vi "test harness_FXP_L_ye_Bend_u_singleAxis.vi"(8 "error in (no error)":errorcluster, 11 "TestCase in":refnum<class "FXP_observer_TestCase.lvclass">) -> (0 "error out":errorcluster, 3 "TestCase out":refnum<class "FXP_observer_TestCase.lvclass">)   [LabVIEW 2017, in "FXP_observer_TestCase.lvclass"]
uses:
  FXP_observer_TestCase.lvclass
  <vilib>/rvi/DesktopExecutionNode/Execution/niFpgaDEN_Execute.vi
  <vilib>/rvi/DesktopExecutionNode/DesktopExecutionNode.xnode
  <vilib>/addons/_JKI Toolkits/VI Tester/TestCase.llb/TestCase.lvclass
  C:/Program Files (x86)/National Instruments/LabVIEW 2017/vi.lib/addons/_JKI Toolkits/VI Tester/TestCase.llb/TestCase.lvclass
panel:
  out "x+y":fxp<+/-,51,11>[](array[numeric])
  out "xk_1_1":fxp<+/-,32,5>[](array[numeric])
  out "error (x_1_1)":errorcluster
  out "error (xu)":errorcluster
  out "error (yd)":errorcluster
  in  "x_u(k)":fxp<+/-,32,8>=13.600000023841858
  in  "Bz":fxp<+/-,32,5>[](array[numeric])=[1.0, 0.5, 0.20000000298023224, 0.20000000298023224, 0.29999999701976776, 2.0, 0.0, 0.0, 0.0, 0.0, 0.0, 0.0, 0.0, 0.0, 0.0, 0.0, 0.0, 0.0, 0.0, 0.0, 0.0, 0.0, 0.0, 0.0, 0.0, 0.0, 0.0, 0.0, 0.0, 0.0, 0.0, 0.0, 0.0, 0.0, 0.0, 0.0, 0.0, 0.0, 0.0, 0.0, 0.0, 0.0, 0.0, 0.0, 0.0, 0.0, 0.0, 0.0, 0.0, 0.0]
  in  "U(k): ux":fxp<+/-,18,5>=0.14501953125
  in  "y(k)":fxp<+/-,18,5>=0.123046875
  in  "NS":u8=5
  in  "Ldist":fxp<+/-,32,5>[](array[numeric])=[1.0, 0.5, 0.20000000298023224, 0.20000000298023224, 0.29999999701976776, 2.0, 0.0, 0.0, 0.0, 0.0, 0.0, 0.0, 0.0, 0.0, 0.0, 0.0, 0.0, 0.0, 0.0, 0.0, 0.0, 0.0, 0.0, 0.0, 0.0, 0.0, 0.0, 0.0, 0.0, 0.0, 0.0, 0.0, 0.0, 0.0, 0.0, 0.0, 0.0, 0.0, 0.0, 0.0, 0.0, 0.0, 0.0, 0.0, 0.0, 0.0, 0.0, 0.0, 0.0, 0.0]
  in  "x":fxp<+/-,32,5>[](array[numeric])=[1.0, 2.0, 3.0, 4.0, 5.0, 2.0, 0.0, 0.0, 0.0, 0.0, 0.0, 0.0, 0.0, 0.0, 0.0, 0.0, 0.0, 0.0, 0.0, 0.0, 0.0, 0.0, 0.0, 0.0, 0.0, 0.0, 0.0, 0.0, 0.0, 0.0, 0.0, 0.0, 0.0, 0.0, 0.0, 0.0, 0.0, 0.0, 0.0, 0.0, 0.0, 0.0, 0.0, 0.0, 0.0, 0.0, 0.0, 0.0, 0.0, 0.0]
  # "Remember that Ldist and Bz only have\ntwo integer bits!"
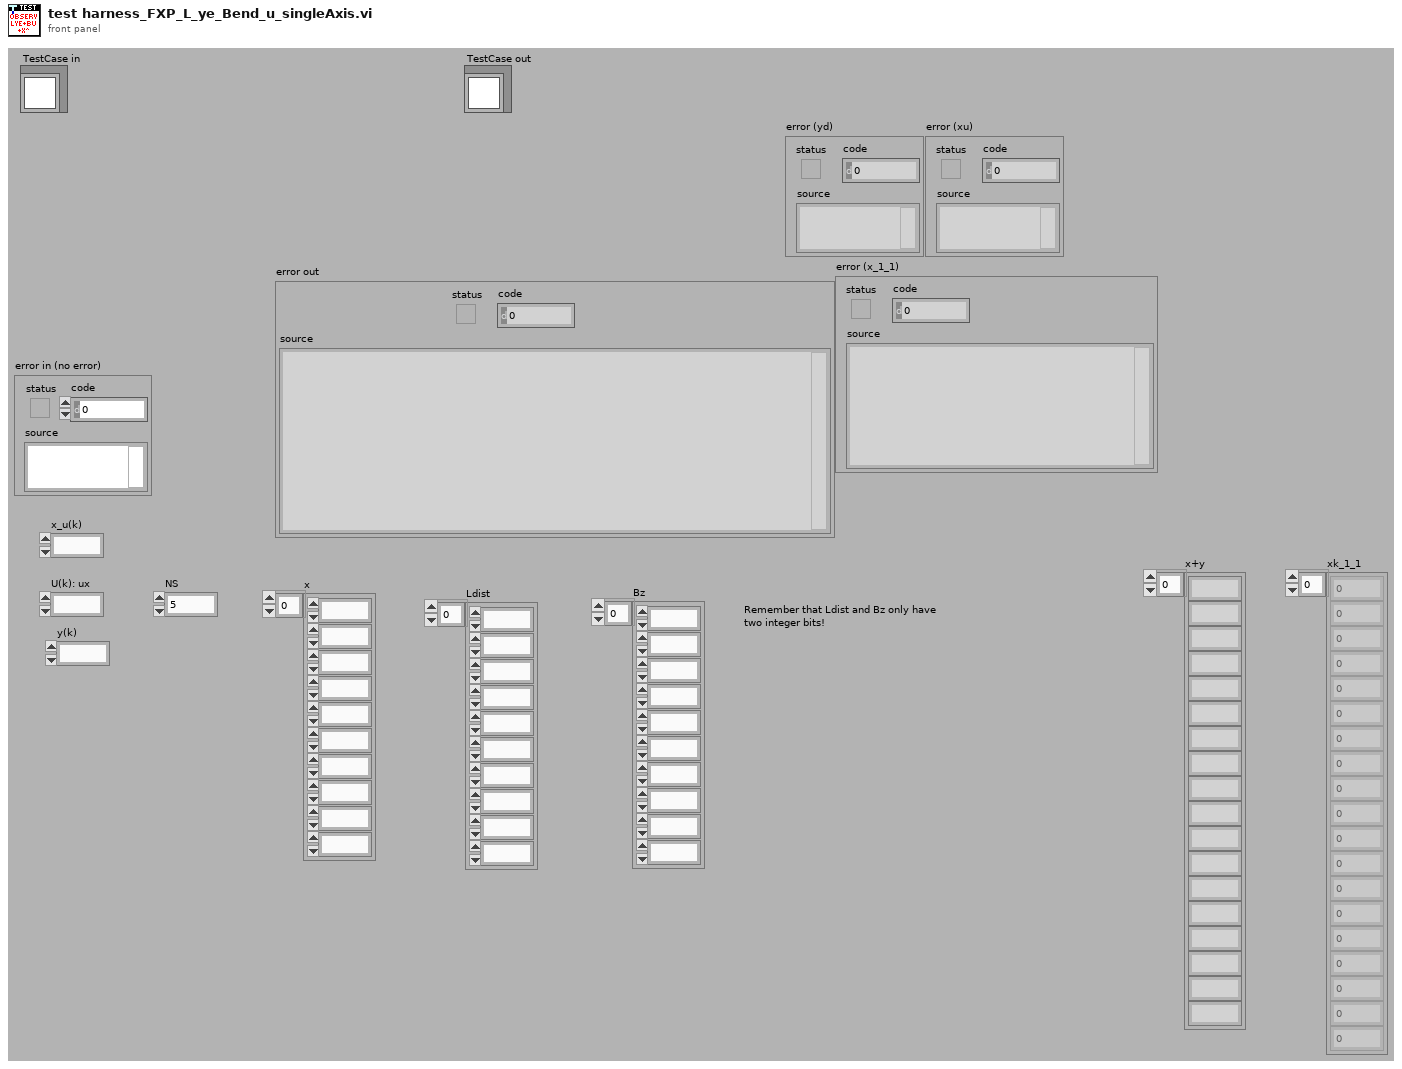
[diagram p1: front panel]
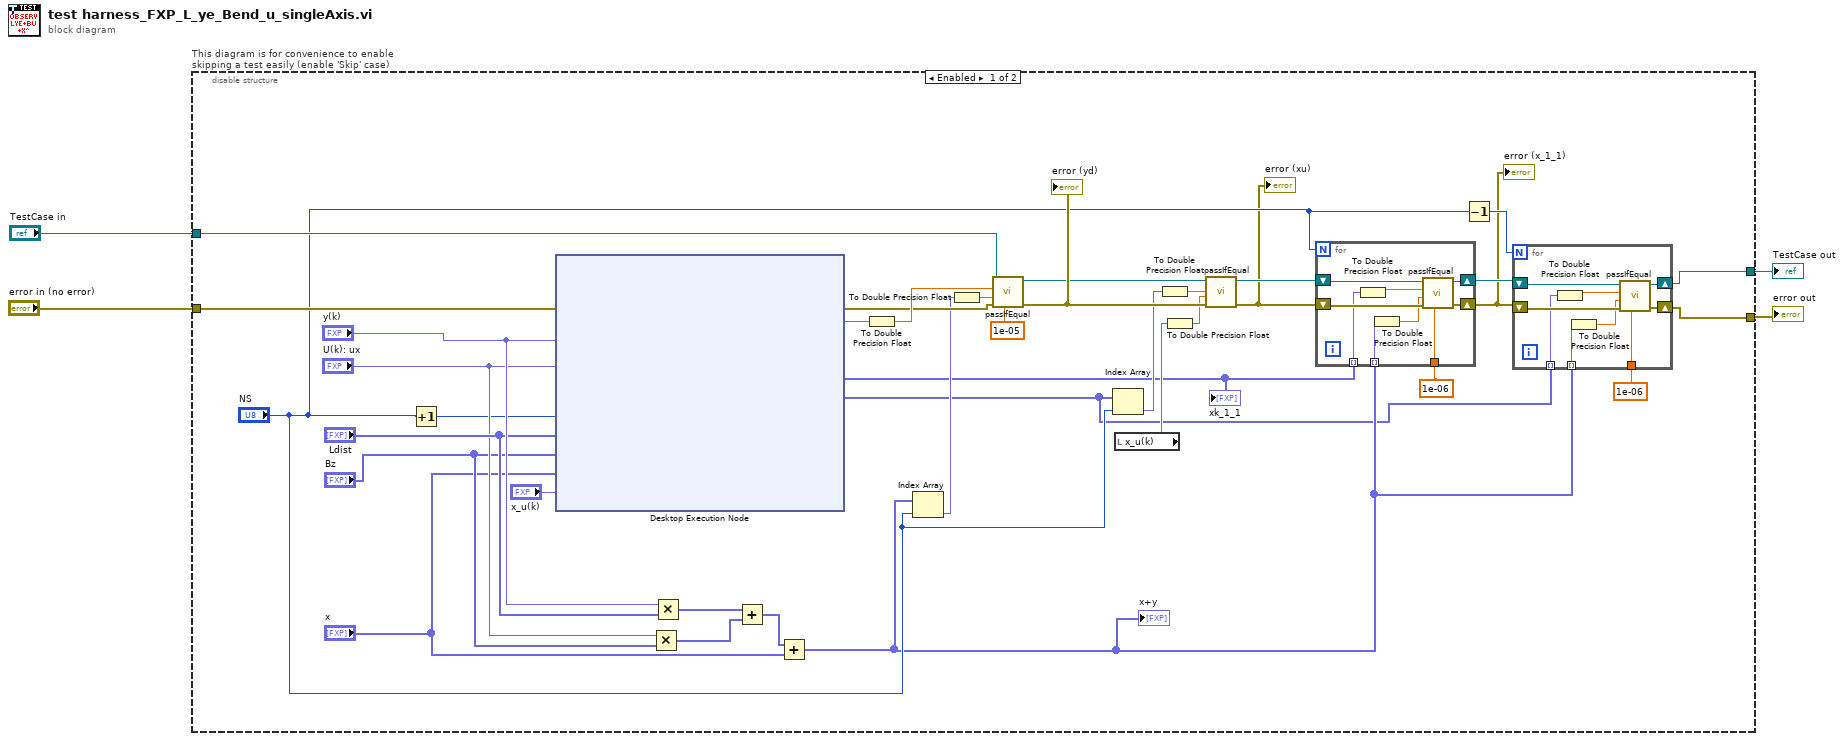
[diagram p0: block diagram]
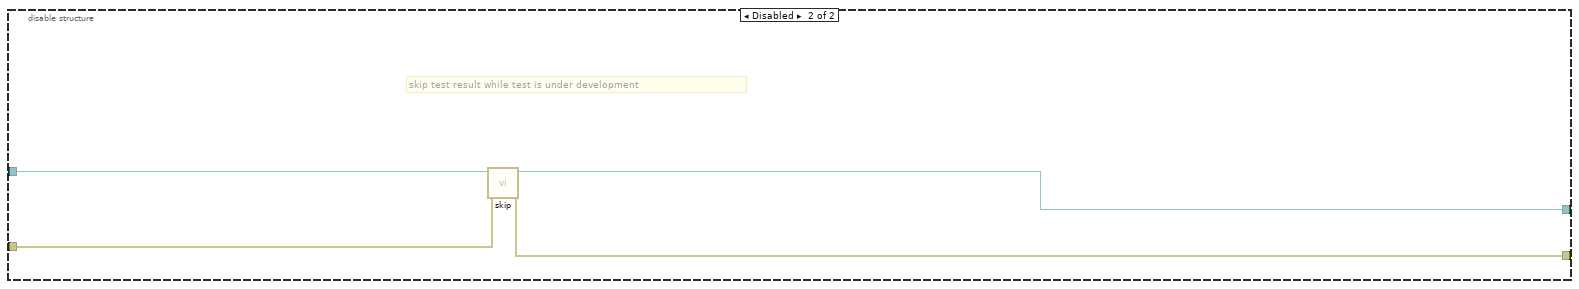
[diagram p2: hidden frame]
diagram:
  n1 = disable-structure "This diagram is for convenience to enable skipping a test easily (enable 'Skip' case)" shown="Enabled" {
    disable-tunnel: "TestCase in" -> [w41 w63]
    disable-tunnel: [w13 w61] -> w1
    disable-tunnel: [w12 w62] -> w3
    disable-tunnel: "error in (no error)" -> [w37 w60]
    frame Enabled {
      n2 = Increment(x="NS") -> (x+1=w25:u8)
      n3 = xnode "Desktop Execution Node"("Error In"=w37, "y(k)"="y(k)", "U(k): ux"="U(k): ux", "NS + 1"=w25, "Ldist"="Ldist", "Bz"="Bz", "x"="x", "x_u(k)"="x_u(k)") -> ("Error Out"=w38:errorcluster, "yd_est"=w28:fxp<+/-,32,5>, "xk_1_1"=w16:fxp<+/-,32,5>[], "xk_1_2"=w7:fxp<+/-,32,5>[])
      "xk_1_1" <- w16
      n4 = Multiply(x="U(k): ux", y="Bz") -> (x*y=w31:fxp<+/-,50,10>[])
      n5 = Multiply(x="y(k)", y="Ldist") -> (x*y=w32:fxp<+/-,50,10>[])
      n6 = Add(x=w32, y=w31) -> (x+y=w30:fxp<+/-,51,11>[])
      n7 = Add(x=w30, y="x") -> (x+y=w8:fxp<+/-,51,11>[])
      "x+y" <- w8
      n8 = To Double Precision Float(number=w28) -> (double precision float=w39:dbl)
      n9 = Index Array(array=w8, index="NS") -> (element=w26:fxp<+/-,51,11>)
      n10 = To Double Precision Float(number=w26) -> (double precision float=w27:dbl)
      n11 = call-dynamic "passIfEqual.vi"("delta (optional)"=1e-05 ("del u_x"), "error in (no error)"=w38, "y"=w27, "x"=w39, "TestCase in"=w41) -> ("error out"=w23:errorcluster, "TestCase out"=w22:refnum<class "FXP_observer_TestCase.lvclass">)  [unwired: 5 in]
      "error (yd)" <- w23
      n12 = Index Array(array=w7, index="NS") -> (element=w20:fxp<+/-,32,5>)
      n13 = local read "x_u(k)"() -> (w18:fxp<+/-,32,8>)
      n14 = To Double Precision Float(number=w20) -> (double precision float=w21:dbl)
      n15 = To Double Precision Float(number=w18) -> (double precision float=w19:dbl)
      n16 = call-dynamic "passIfEqual.vi"("error in (no error)"=w23, "y"=w19, "x"=w21, "TestCase in"=w22) -> ("error out"=w6:errorcluster, "TestCase out"=w17:refnum<class "FXP_observer_TestCase.lvclass">)  [unwired: 6 in]
      "error (xu)" <- w6
      n17 = for {
        N: "NS" -> [_]
        shift-right: [w59] -> w14
        shift-left: w17 -> [w56]
        shift-right: [w58] -> w5
        shift-left: w6 -> [w57]
        tunnel: w8 -> [w55] mode=indexing
        tunnel: w16 -> [w52] mode=indexing
        tunnel: 1e-06 ("del u_x") -> [w51]
        n18 = To Double Precision Float(number=w52) -> (double precision float=w53:dbl)
        n19 = To Double Precision Float(number=w55) -> (double precision float=w54:dbl)
        n20 = call-dynamic "passIfEqual.vi"("delta (optional)"=w51, "error in (no error)"=w57, "y"=w54, "x"=w53, "TestCase in"=w56) -> ("error out"=w58:errorcluster, "TestCase out"=w59:refnum<class "FXP_observer_TestCase.lvclass">)  [unwired: 5 in]
      }
      "error (x_1_1)" <- w5
      n21 = Decrement(x="NS") -> (x-1=w10:u8)
      n22 = for {
        N: w10 -> [_]
        shift-right: [w50] -> w13
        shift-left: w14 -> [w47]
        shift-right: [w49] -> w12
        shift-left: w5 -> [w48]
        tunnel: w8 -> [w46] mode=indexing
        tunnel: w7 -> [w43] mode=indexing
        tunnel: 1e-06 ("del u_x") -> [w42]
        n23 = To Double Precision Float(number=w43) -> (double precision float=w44:dbl)
        n24 = To Double Precision Float(number=w46) -> (double precision float=w45:dbl)
        n25 = call-dynamic "passIfEqual.vi"("delta (optional)"=w42, "error in (no error)"=w48, "y"=w45, "x"=w44, "TestCase in"=w47) -> ("error out"=w49:errorcluster, "TestCase out"=w50:refnum<class "FXP_observer_TestCase.lvclass">)  [unwired: 5 in]
      }
    }
    frame Disabled {
      # "skip test result while test is under development"
      n26 = call <vilib>:"skip.vi"("error in (no error)"=w60, "TestCase in"=w63) -> ("error out"=w62:errorcluster, "TestCase out"=w61:refnum<class "FXP_observer_TestCase.lvclass">)  [unwired: 8 in]
    }
  }
  "error out" <- w3
  "TestCase out" <- w1
